vi "ClimbBegin.vi"(8 "error in (no error)":errorcluster) -> (0 "error out":errorcluster)   [LabVIEW 2023]
uses:
  <vilib>/Rock Robotics/WPI/ThirdParty/REV Robotics/REVLib/Typedef/Spark MAX Limit Switch Polarity.ctl
  <vilib>/Rock Robotics/WPI/ThirdParty/REV Robotics/REVLib/Typedef/Spark MAX Limit Direction.ctl
  <vilib>/Rock Robotics/WPI/ThirdParty/REV Robotics/REVLib/Typedef/Spark MAX Idle Mode.ctl
  <vilib>/Rock Robotics/WPI/ThirdParty/REV Robotics/REVLib/Typedef/Spark MAX Motor Type.ctl
  <vilib>/Rock Robotics/WPI/ThirdParty/REV Robotics/REVLib/Typedef/Spark MAX Sensor Type.ctl
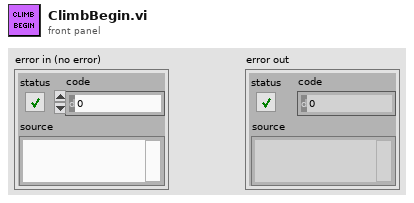
[diagram p1: front panel]
types:
  T1 = typedef "Spark MAX Sensor Type.ctl" = enum16{"No Sensor", "Hall Sensor", "Encoder", "-Not Available-", "Analog", "Alternate Encoder", "Duty Cycle"}
  T2 = typedef "Spark MAX Limit Switch Polarity.ctl" = enum16{"Normally Open", "Normally Closed"}
  T3 = typedef "Spark MAX Limit Direction.ctl" = enum16{"Forward Limit", "Reverse Limit"}
  T4 = typedef "Spark MAX Idle Mode.ctl" = enum16{"Coast", "Brake"}
  T5 = typedef "Spark MAX Motor Type.ctl" = enum16{"Brushed", "Brushless"}
  T6 = typedef "WPI_MotorControlDeviceRef.ctl" = cluster{"DeviceStatus":errorcluster, "Type":T7, "PWM":cluster{"PWM Channel":T8, "DeadBand":T9}, "CAN":cluster{"Device Number":u8, "SetOutput VI Ref":variant, "GetOutput VI Ref":variant, "Enable VI Ref":variant, "Disable VI Ref":variant, "Data":variant}, "Invert":bool, "DIO PWM":cluster{"PWM \"Enable\" Channel":T8, "DIOChannel":T10, "PWM Rate":dbl}}
  T7 = typedef "WPI_MotorControlType.ctl" = enum16{"PWM", "CAN", "DIO PWM"}
  T8 = typedef "FPGA_DIOPWMChannel.ctl" = enum8{"PWM 0", "PWM 1", "PWM 2", "PWM 3", "PWM 4", "PWM 5", "PWM 6", "PWM 7", "PWM 8", "PWM 9", "PWM MXP 0", "PWM MXP 1", "PWM MXP 2", "PWM MXP 3", "PWM MXP 4", "PWM MXP 5", "PWM MXP 6", "PWM MXP 7", "PWM MXP 8", "PWM MXP 9", "Invalid"}
  T9 = typedef "WPI_PWMDeadband.ctl" = cluster{"Name":string, "maxPositivePwm":i32, "minPositivePwm":i32, "centerPwm":i32, "maxNegativePwm":i32, "minNegativePwm":i32, "angularRange":u16}
  T10 = typedef "FPGA_DIOChannel.ctl" = enum8{"DIO 0", "DIO 1", "DIO 2", "DIO 3", "DIO 4", "DIO 5", "DIO 6", "DIO 7", "DIO 8", "DIO 9", "DIO MXP 0", "DIO MXP 1", "DIO MXP 2", "DIO MXP 3", "DIO MXP 4", "DIO MXP 5", "DIO MXP 6", "DIO MXP 7", "DIO MXP 8", "DIO MXP 9", "DIO MXP 10", "DIO MXP 11", "DIO MXP 12", "DIO MXP 13", "DIO MXP 14", "DIO MXP 15", "SPI Port CS1", "SPI Port CS2", "SPI Port CS3", "SPI Port MISO", "SPI Port MOSI", "Invalid"}
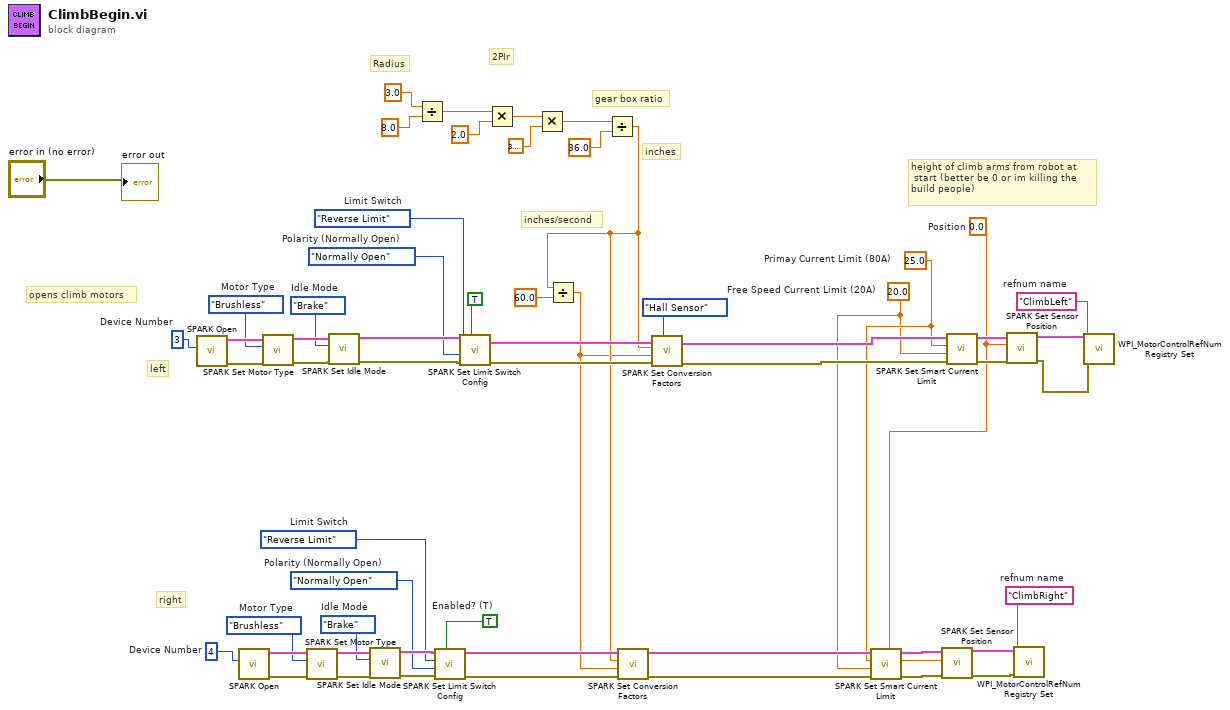
[diagram p0: block diagram]
diagram:
  w7 = 0.0  # Position
  w25 = TRUE  # Enabled? (T)
  w2 = 20.0  # Free Speed Current Limit (20A)
  w3 = 25.0  # Primay Current Limit (80A)
  w27 = Spark_MAX_Limit_Switch_Polarity."Normally Open"  # Polarity (Normally Open)
  w28 = Spark_MAX_Limit_Direction."Reverse Limit"  # Limit Switch
  w29 = Spark_MAX_Limit_Switch_Polarity."Normally Open"  # Polarity (Normally Open)
  w30 = Spark_MAX_Limit_Direction."Reverse Limit"  # Limit Switch
  w40 = Spark_MAX_Idle_Mode."Brake"  # Idle Mode
  w41 = Spark_MAX_Idle_Mode."Brake"  # Idle Mode
  w44 = Spark_MAX_Motor_Type."Brushless"  # Motor Type
  w45 = Spark_MAX_Motor_Type."Brushless"  # Motor Type
  w46 = "ClimbRight"  # refnum name
  w47 = "ClimbLeft"  # refnum name
  w51 = u8 4  # Device Number
  w52 = u8 3  # Device Number
  # "inches/second"
  # "inches"
  # "height of climb arms from robot at\n start (better be 0 or im killing the \nbuild people)"
  # "gear box ratio"
  # "2PIr"
  # "Radius"
  # "opens climb motors"
  # "right"
  # "left"
  n1 = call <vilib>:"SPARK Open.vi"("Device Number"=w52) -> ("error out"=w53:errorcluster, "MotorControlDeviceRef"=w54:T6)  [unwired: 9 in]
  n2 = call <vilib>:"SPARK Open.vi"("Device Number"=w51) -> ("error out"=w37:errorcluster, "MotorControlDeviceRef"=w50:T6)  [unwired: 9 in]
  n3 = call <vilib>:"SPARK Set Motor Type.vi"("error in (no error)"=w53, "Motor Type"=w45, "MotorControlDevRef"=w54) -> ("error out"=w39:errorcluster, "MotorControlDeviceRef"=w43:T6)  [unwired: 7 in]
  n4 = call <vilib>:"SPARK Set Motor Type.vi"("error in (no error)"=w37, "Motor Type"=w44, "MotorControlDevRef"=w50) -> ("error out"=w36:errorcluster, "MotorControlDeviceRef"=w42:T6)  [unwired: 7 in]
  n5 = call <vilib>:"SPARK Set Idle Mode.vi"("error in (no error)"=w39, "Idle Mode"=w40, "MotorControlDeviceRef in"=w43) -> ("error out"=w31:errorcluster, "MotorControlDeviceRef out"=w32:T6)  [unwired: 7 in]
  n6 = call <vilib>:"SPARK Set Idle Mode.vi"("error in (no error)"=w36, "Idle Mode"=w41, "MotorControlDeviceRef in"=w42) -> ("error out"=w33:errorcluster, "MotorControlDeviceRef out"=w34:T6)  [unwired: 7 in]
  n7 = Divide(x=3.0, y=8.0) -> (x/y=w17:dbl)
  n8 = call <vilib>:"SPARK Set Limit Switch Config.vi"("Enabled? (T)"=w25, "error in (no error)"=w33, "Polarity (Normally Open)"=w27, "Limit Switch"=w28, "MotorControlDeviceRef in"=w34) -> ("error out"=w9:errorcluster, "MotorControlDeviceRef out"=w11:T6)  [unwired: 5 in]
  n9 = call <vilib>:"SPARK Set Limit Switch Config.vi"("Enabled? (T)"=TRUE, "error in (no error)"=w31, "Polarity (Normally Open)"=w29, "Limit Switch"=w30, "MotorControlDeviceRef in"=w32) -> ("error out"=w22:errorcluster, "MotorControlDeviceRef out"=w24:T6)  [unwired: 5 in]
  n10 = Multiply(x=w17, y=2.0) -> (x*y=w15:dbl)
  n11 = Multiply(x=w15, y=3.141592653589793) -> (x*y=w13:dbl)
  n12 = Divide(x=w13, y=36.0) -> (x/y=w5:dbl)
  n13 = Divide(x=w5, y=60.0) -> (x/y=w4:dbl)
  n14 = call <vilib>:"SPARK Set Conversion Factors.vi"("error in (no error)"=w9, "Velocity Factor (1)"=w4, "Position Factor (1)"=w5, "MotorControlDeviceRef in"=w11) -> ("error out"=w8:errorcluster, "MotorControlDeviceRef out"=w10:T6)  [unwired: 6 in]
  n15 = call <vilib>:"SPARK Set Conversion Factors.vi"("Sensor Type (Hall Sensor)"=Spark_MAX_Sensor_Type."Hall Sensor", "error in (no error)"=w22, "Velocity Factor (1)"=w4, "Position Factor (1)"=w5, "MotorControlDeviceRef in"=w24) -> ("error out"=w21:errorcluster, "MotorControlDeviceRef out"=w23:T6)  [unwired: 5 in]
  n16 = call <vilib>:"SPARK Set Smart Current Limit.vi"("error in (no error)"=w8, "Free Speed Current Limit (20A)"=w2, "Primay Current Limit (80A)"=w3, "MotorControlDeviceRef in"=w10) -> ("error out"=w56:errorcluster, "MotorControlDeviceRef out"=w55:T6)  [unwired: 6 in]
  n17 = call <vilib>:"SPARK Set Sensor Position.vi"("error in"=w56, "Position"=w7, "MotorControlDeviceRef"=w55) -> ("error out"=w35:errorcluster, "MotorControlDeviceRef"=w48:T6)  [unwired: 7 in]
  n18 = call <vilib>:"SPARK Set Smart Current Limit.vi"("error in (no error)"=w21, "Free Speed Current Limit (20A)"=w2, "Primay Current Limit (80A)"=w3, "MotorControlDeviceRef in"=w23) -> ("error out"=w58:errorcluster, "MotorControlDeviceRef out"=w57:T6)  [unwired: 6 in]
  n19 = call <vilib>:"SPARK Set Sensor Position.vi"("error in"=w58, "Position"=w7, "MotorControlDeviceRef"=w57) -> ("error out"=w38:errorcluster, "MotorControlDeviceRef"=w49:T6)  [unwired: 7 in]
  n20 = call <vilib>:"WPI_MotorControlRefNum Registry Set.vi"("error in (no error)"=w35, "refnum name"=w46, "MotorControlDevRef"=w48) -> ()  [unwired: 7 in, 2 out]
  n21 = call <vilib>:"WPI_MotorControlRefNum Registry Set.vi"("error in (no error)"=w38, "refnum name"=w47, "MotorControlDevRef"=w49) -> ()  [unwired: 7 in, 2 out]
  "error out" <- "error in (no error)"
